vi "Main.vi"(8 "error in":errorcluster, 11 "Listener in":refnum<class "Listener.lvclass">) -> (0 "error out":errorcluster, 3 "Listener out":refnum<class "Listener.lvclass">)   [LabVIEW 2020, in "Listener.lvclass"]
doc: "The Queued Message Handler of a Worker."
uses:
  Listener.lvclass
  C:/Program Files (x86)/National Instruments/LabVIEW 2020/vi.lib/addons/_Workers/Library/Classes/Worker/Worker.lvclass
  Initialization Data.ctl
  Listener.lvclass/Listener.ctl
  <vilib>/addons/_Workers/Library/Classes/Message/Enqueue Message to Self.vi
  <vilib>/addons/_Workers/Library/Classes/Message/Enqueue Message to Queue.vi
  <vilib>/addons/_Workers/Library/Classes/EHL/EHL.lvclass
  <vilib>/addons/_Workers/Library/Classes/Worker/Worker.lvclass
  <vilib>/addons/_Workers/Library/Classes/Error Handler/Error Handler.lvclass
  C:/Program Files (x86)/National Instruments/LabVIEW 2020/vi.lib/addons/_Workers/Library/Classes/Worker User/Worker User.lvclass
  C:/Program Files (x86)/National Instruments/LabVIEW 2020/vi.lib/addons/_Workers/Library/Classes/Workers Object/Workers Object.lvclass
  C:/Users/TestAdmin/git/TCP-Workers/Workers/Listener/Listener.lvclass
  <vilib>/addons/_Workers/Library/Classes/Message/Message.lvclass
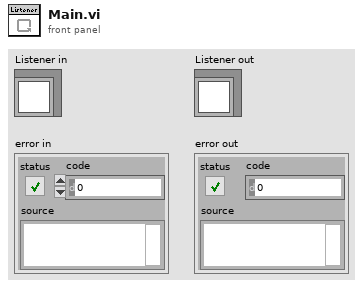
[diagram p1: front panel]
types:
  T1 = typedef "Listener.lvclass/Initialization Data.ctl" = cluster{"String":string, "port":u16}
  T2 = typedef "Workers.lvlib/Case Label.ctl" = string
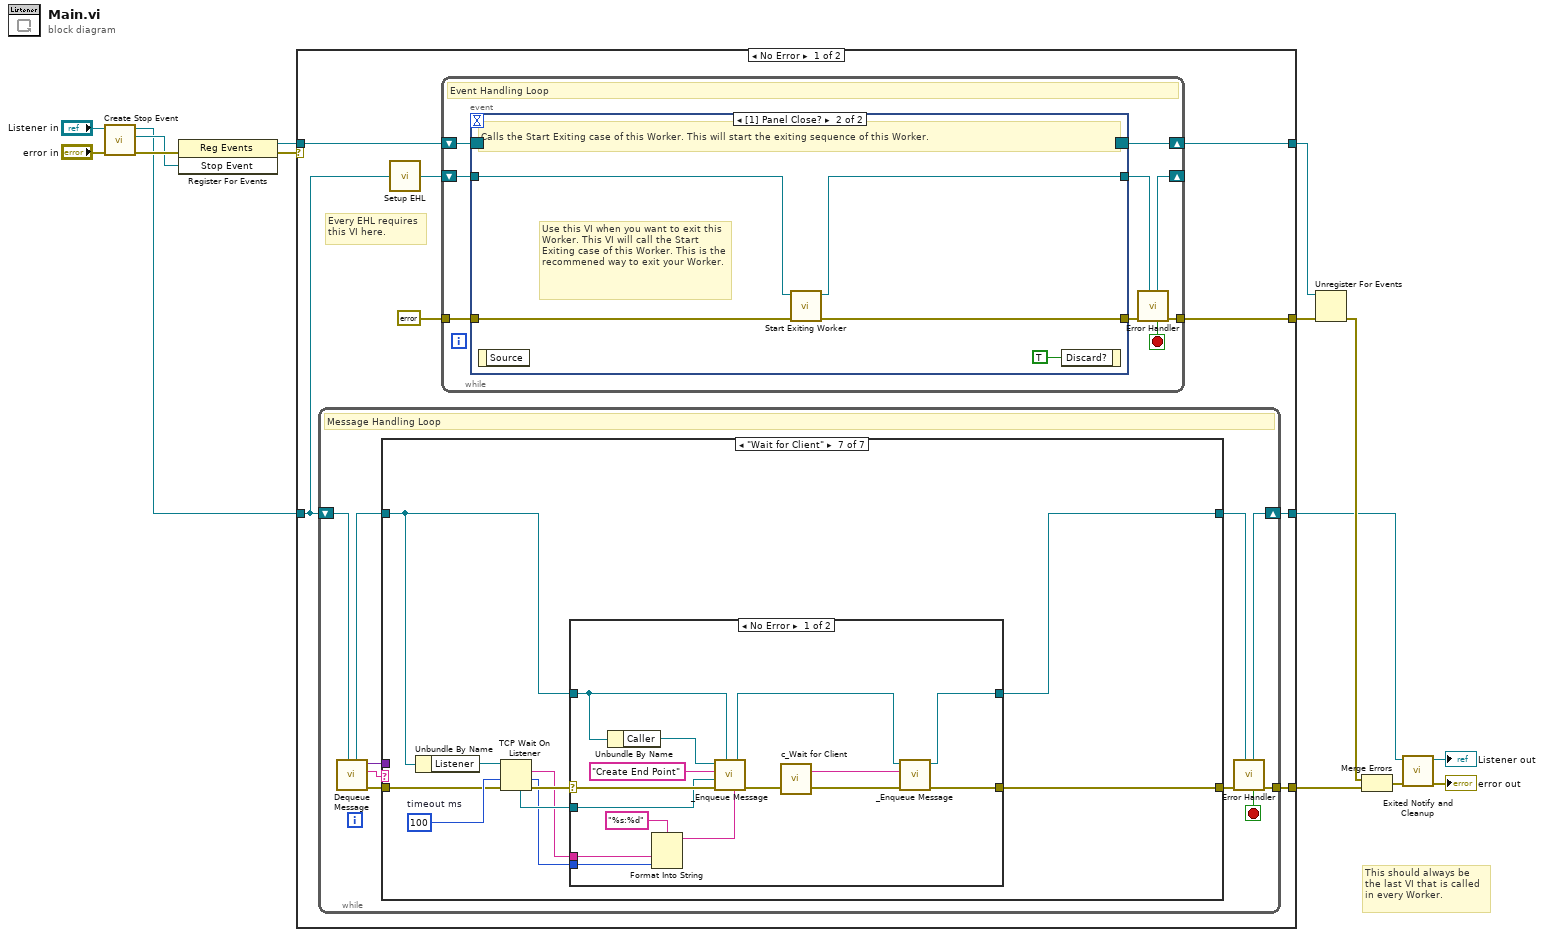
[diagram p0: block diagram]
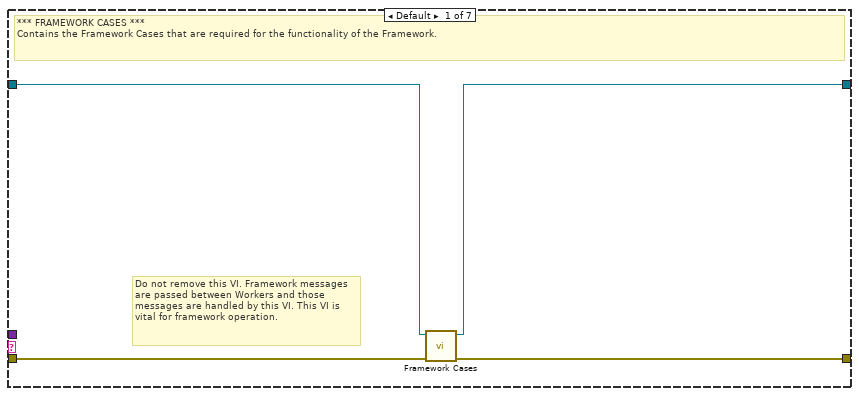
[diagram p2: hidden frame]
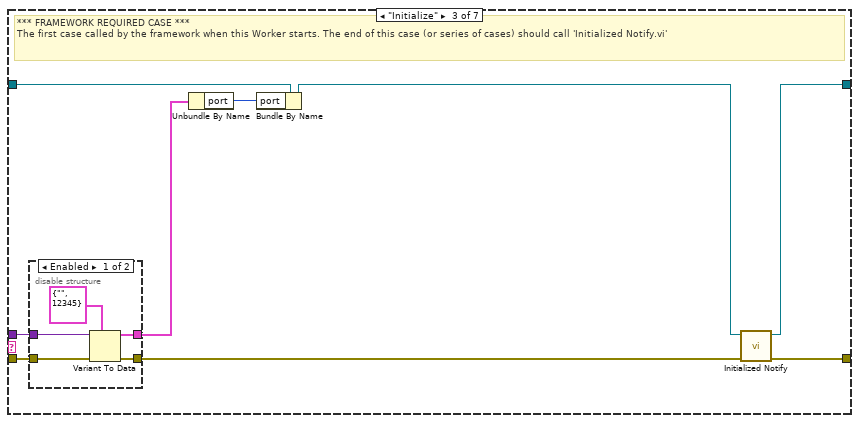
[diagram p4: hidden frame]
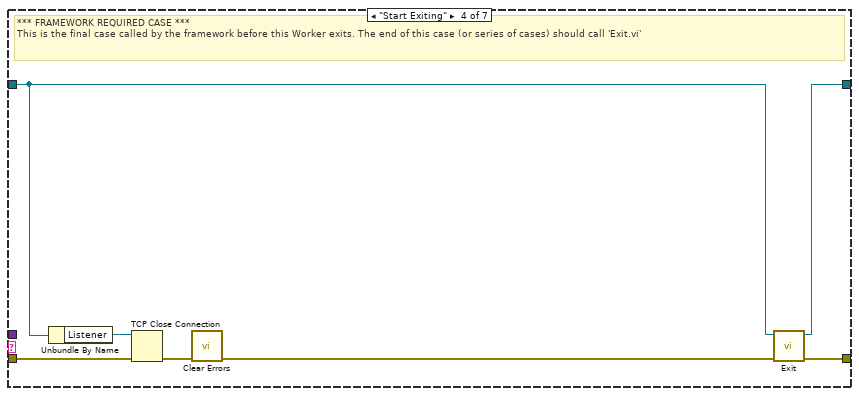
[diagram p6: hidden frame]
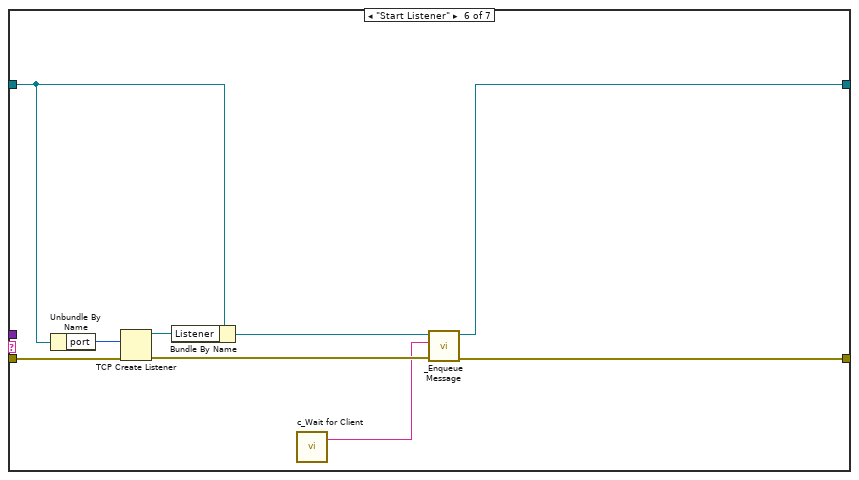
[diagram p8: hidden frame]
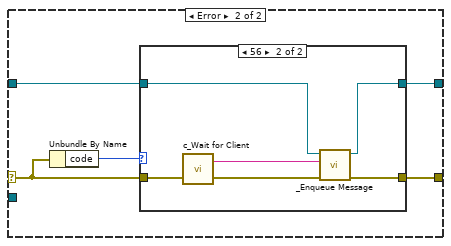
[diagram p9: hidden frame]
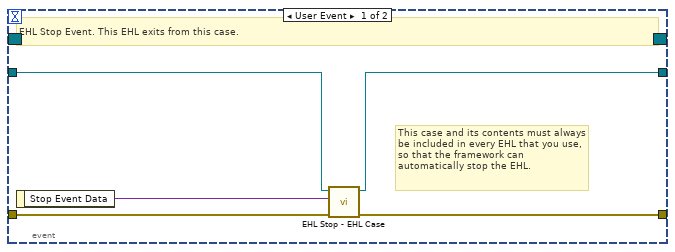
[diagram p11: hidden frame]
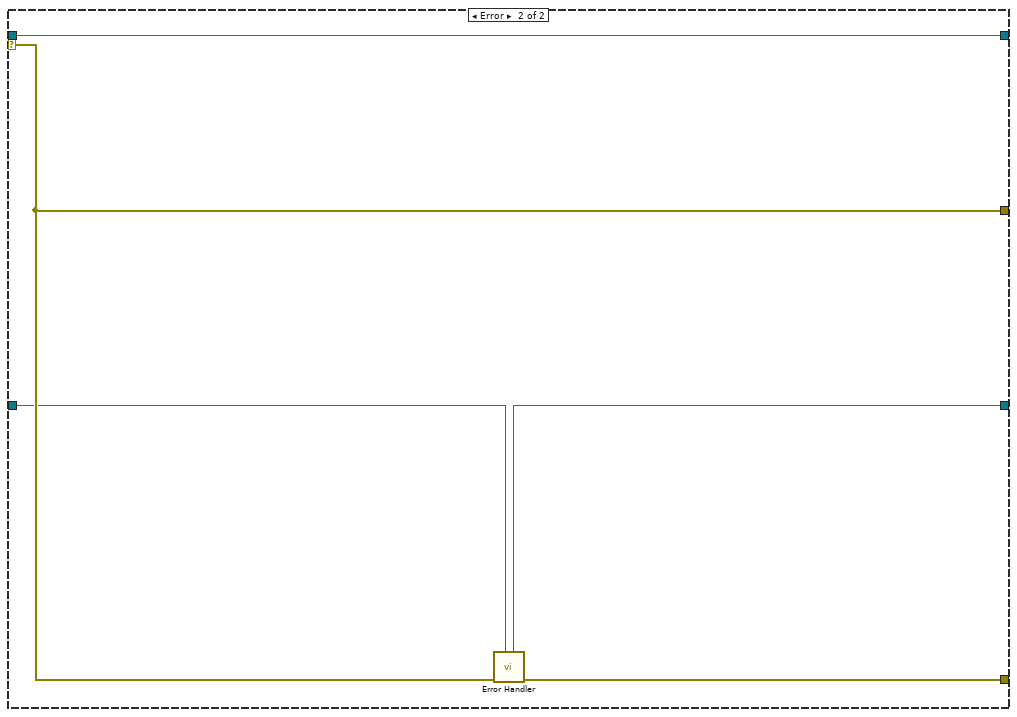
[diagram p12: hidden frame]
diagram:
  # "This should always be the last VI that is called in every Worker."
  n1 = call <vilib>:"Create Stop Event.vi"("error in"="error in", "Worker"="Listener in") -> ("error out"=w10:errorcluster, "Stop Event"=w7:refnum<user-event>, "Worker out"=w4:refnum<class "Listener.lvclass">)  [unwired: 7 in]
  n2 = register-events(error in=w10, w7) -> (reference out=w9:refnum<event-registration>, error out=w1:errorcluster)  [unwired: 1 in]
  n3 = case shown="No Error" w1 {
    tunnel: w4 -> [w18 w129]
    tunnel: [w16 w130] -> w8
    tunnel: w9 -> [w23 w131]
    tunnel: [w20 w132] -> w14
    tunnel: [w22 w131] -> w13
    tunnel: [w17 w128] -> w11
    selector: w1 -> [_ w132]
    frame No Error {
      # "Every EHL requires\nthis VI here."
      n4 = while {
        shift-right: [w31] -> w17
        shift-left: w18 -> [w33]
        tunnel: [w32] -> w16
        stop <- w24 stop-if-true
        # "Message Handling Loop"
        n5 = call <vilib>:"Dequeue Message.vi"("Worker"=w33) -> ("error out"=w30:errorcluster, "Case out"=w25:string, "Data out"=w26:variant, "Worker out"=w28:refnum<class "Listener.lvclass">)  [unwired: 6 in, 1 out]
        n6 = case "WORKERS MHL Case Structure (DO NOT CHANGE LABEL NAME)" shown="\"Wait for Client\"" w25 {
          tunnel: w30 -> [w37 w38 w46 w59 w62 w72 w81]
          tunnel: [w36 w38 w48 w61 w62 w65 w76] -> w29
          tunnel: w28 -> [w35 w39 w45 w58 w63 w71 w78]
          tunnel: [w34 w39 w47 w60 w63 w66 w75] -> w27
          tunnel: w26 -> [_ _ w43 _ _ _ _]
          frame Default {
            # "Do not remove this VI. Framework messages are passed between Workers and those messages are handled by this VI. This VI is vital for framework operation."
            # "*** FRAMEWORK CASES ***\nContains the Framework Cases that are required for the functionality of the Framework."
            n7 = call <vilib>:"Framework Cases.vi"("error in"=w37, "Worker"=w35) -> ("error out"=w36:errorcluster, "Worker out"=w34:refnum<class "Listener.lvclass">)  [unwired: 8 in]
          }
          frame "------ FRAMEWORK REQUIRED CASES ------" {
            # "Start of Framework Required Cases"
          }
          frame "Initialize" {
            # "*** FRAMEWORK REQUIRED CASE ***\nThe first case called by the framework when this Worker starts. The end of this case (or series of cases) should call 'Initialized Notify.vi'"
            n8 = disable-structure shown="Enabled" {
              disable-tunnel: w46 -> [w53 w54]
              disable-tunnel: [w52 w54] -> w44
              disable-tunnel: w43 -> [w51 _]
              disable-tunnel: [w49 _] -> w41
              frame Enabled {
                n9 = Variant To Data(error in=w53, type=T1 {"String"="", "port"=12345} ("Initialization Data"), Variant=w51) -> (data=w49:T1, error out=w52:errorcluster)
              }
              frame Disabled {
              }
            }
            n10 = Unbundle By Name(w41) -> ("port"=w40:u16)
            n11 = Bundle By Name(cluster=w45, "port"=w40) -> (w42:refnum<class "Listener.lvclass">)
            n12 = call <vilib>:"Initialized Notify.vi"("error in"=w44, "Worker"=w42) -> ("error out"=w48:errorcluster, "dup Worker out"=w47:refnum<class "Listener.lvclass">)  [unwired: 8 in]
          }
          frame "Start Exiting" {
            # "*** FRAMEWORK REQUIRED CASE ***\nThis is the final case called by the framework before this Worker exits. The end of this case (or series of cases) should call 'Exit.vi'"
            n13 = Unbundle By Name(w58) -> ("Listener"=w57:refnum<k5>)
            n14 = TCP Close Connection(connection ID=w57, error in (no error)=w59) -> (error out=w56:errorcluster)  [unwired: 1 in, 1 out]
            n15 = call <vilib>:"Clear Errors.vi"("error in (no error)"=w56) -> ("error out"=w55:errorcluster)  [unwired: 5 in, 1 out]
            n16 = call <vilib>:"Exit.vi"("error_in"=w55, "Worker"=w58) -> ("error out"=w61:errorcluster, "dup Worker out"=w60:refnum<class "Listener.lvclass">)  [unwired: 8 in]
          }
          frame "-----------------------------------------------" {
            # "End of Framework Required Cases"
          }
          frame "Start Listener" {
            n17 = Unbundle By Name(w71) -> ("port"=w70:u16)
            n18 = TCP Create Listener(8:w72, 10:w70) -> (0:w68:errorcluster, 3:w69:refnum<k5>)  [unwired: 4 out]
            n19 = Bundle By Name(cluster=w71, "Listener"=w69) -> (w67:refnum<class "Listener.lvclass">)
            n20 = call "c_Wait for Client.vi"() -> ("Case Label"=w64:T2)  [unwired: 1 in]
            n21 = call-poly <vilib>:"_Enqueue Message.vi"("error in"=w68, "Case Label"=w64, "Worker"=w67) -> ("error out"=w65:errorcluster, "dup Worker out"=w66:refnum<class "Listener.lvclass">)  [unwired: 7 in]
          }
          frame "Wait for Client" {
            w82 = 100  # timeout ms
            n22 = Unbundle By Name(w78) -> ("Listener"=w80:refnum<k5>)
            n23 = TCP Wait On Listener(8:w81, 9:w82, 11:w80) -> (0:w79:errorcluster, 1:w73:u16, 2:w74:string, 4:w77:refnum<k5>)  [unwired: 2 out]
            n24 = case shown="No Error" w79 {
              selector: w79 -> [w96 w101]
              tunnel: [w91 w99] -> w76
              tunnel: w78 -> [w88 w98]
              tunnel: [w90 w97] -> w75
              tunnel: w77 -> [w95 _]
              tunnel: w74 -> [w84 _]
              tunnel: w73 -> [w83 _]
              frame No Error {
                # "Add the new client connection to the state data and go to the 'Send Data' state."
                n25 = Unbundle By Name(w88) -> ("Caller"=w94:refnum<class "Message Queue.lvclass">)
                n26 = Format Into String(format string="%s:%d", w84, w83) -> (resulting string=w86:string)  [unwired: 2 in, 1 out]
                n27 = call-poly <vilib>:"_Enqueue Message.vi"("Auxiliary"=w86, "Worker"=w88, "error in"=w96, "Data"=w95, "Case Label"="Create End Point", "Message Queue"=w94) -> ("error out"=w92:errorcluster, "dup Worker out"=w87:refnum<class "Listener.lvclass">)  [unwired: 3 in, 1 out]
                n28 = call "c_Wait for Client.vi"() -> ("Case Label"=w89:T2)  [unwired: 1 in]
                n29 = call-poly <vilib>:"_Enqueue Message.vi"("error in"=w92, "Case Label"=w89, "Worker"=w87) -> ("error out"=w91:errorcluster, "dup Worker out"=w90:refnum<class "Listener.lvclass">)  [unwired: 7 in]
              }
              frame Error {
                # "Ignore timeout errors. If there are any clients, go to the 'Send Data' state."
                n30 = Unbundle By Name(w101) -> ("code"=w100:i32)
                n31 = case shown="56" w100 {
                  tunnel: w101 -> [w103 w108]
                  tunnel: [w103 w107] -> w99
                  tunnel: w98 -> [w102 w106]
                  tunnel: [w102 w105] -> w97
                  frame Default {
                  }
                  frame 56 {
                    n32 = call "c_Wait for Client.vi"() -> ("Case Label"=w104:T2)  [unwired: 1 in]
                    n33 = call-poly <vilib>:"_Enqueue Message.vi"("error in"=w108, "Case Label"=w104, "Worker"=w106) -> ("error out"=w107:errorcluster, "dup Worker out"=w105:refnum<class "Listener.lvclass">)  [unwired: 7 in]
                  }
                }
              }
            }
          }
        }
        n34 = call <vilib>:"Error Handler.vi"("Worker"=w27, "error_in"=w29) -> ("error out"=w32:errorcluster, "Stop Loop"=w24:bool, "Worker out"=w31:refnum<class "Listener.lvclass">)  [unwired: 7 in]
      }
      n35 = call <vilib>:"Setup EHL.vi"("Worker"=w18) -> ("Worker out"=w19:refnum<class "Listener.lvclass">)  [unwired: 14 in]
      n36 = while "Event Handling Loop" {
        shift-right: [w117] -> w22
        shift-left: w23 -> [w116]
        tunnel: [w112] -> w20
        tunnel: errorcluster {"status"=FALSE, "code"=0, "source"=""} ("error constant") -> [w114]
        shift-right: [w110] -> _
        shift-left: w19 -> [w115]
        stop <- w109 stop-if-true
        # "Event Handling Loop"
        n37 = event shown="[1] Panel Close?" {
          selector: w116 -> [_ _]
          dyn-events: [_ _] -> w117
          timeout: _ -> [_ _]
          tunnel: [w121 w126] -> w113
          tunnel: w114 -> [w122 w125]
          tunnel: w115 -> [w120 w124]
          tunnel: [w119 w123] -> w111
          event User Event {
            # "This case and its contents must always be included in every EHL that you use, so that the framework can automatically stop the EHL."
            # "EHL Stop Event. This EHL exits from this case."
            n38 = event-data() -> ("Stop Event Data"=w118:variant)  [unwired: 1 in]
            n39 = call <vilib>:"EHL Stop - EHL Case.vi"("error in"=w122, "Stop Event Data"=w118, "Worker"=w120) -> ("error out"=w121:errorcluster, "Worker out"=w119:refnum<class "Listener.lvclass">)  [unwired: 7 in]
          }
          event Panel Close? {
            # "Use this VI when you want to exit this Worker. This VI will call the Start Exiting case of this Worker. This is the recommened way to exit your Worker."
            # "Calls the Start Exiting case of this Worker. This will start the exiting sequence of this Worker."
            n40 = event-data() -> ()  [unwired: 1 in, 1 out]
            n41 = call <vilib>:"Start Exiting Worker.vi"("error in"=w125, "Worker"=w124) -> ("error out"=w126:errorcluster, "dup Worker out"=w123:refnum<class "Listener.lvclass">)  [unwired: 8 in]
            n42 = event-data("Discard?"=TRUE) -> ()  [unwired: 1 in, 1 out]
          }
        }
        n43 = call <vilib>:"Error Handler.vi"("Worker"=w111, "error_in"=w113) -> ("error out"=w112:errorcluster, "Stop Loop"=w109:bool, "Worker out"=w110:refnum<class "Listener.lvclass">)  [unwired: 7 in]
      }
    }
    frame Error {
      n44 = call <vilib>:"Error Handler.vi"("Worker"=w129, "error_in"=w132) -> ("error out"=w130:errorcluster, "Worker out"=w128:refnum<class "Listener.lvclass">)  [unwired: 7 in, 1 out]
    }
  }
  n45 = Unregister For Events(event registration refnum=w13, error in=w14) -> (error out=w15:errorcluster)
  n46 = Merge Errors(w15, w8) -> (w12:errorcluster)
  n47 = call <vilib>:"Exited Notify and Cleanup.vi"("error_in"=w12, "Worker"=w11) -> ("error out"=→"error out":errorcluster, "dup Worker out"=→"Listener out":refnum<class "Listener.lvclass">)  [unwired: 8 in]
